vi "Updater Convert TDMS SP Graphics Channel Groups 4.3 to 5.0.vi"(6 "New TDMS File In":refnum<k34>, 8 "error in (no error)":errorcluster, 10 "Group Name In":string, 11 "Source TDMS File In":refnum<k34>) -> (0 "error out":errorcluster, 2 "Group Name Out":string, 3 "Source TDMS File Out":refnum<k34>, 4 "New TDMS File Out":refnum<k34>)   [LabVIEW 2011]
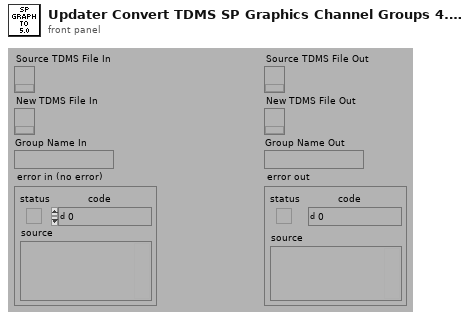
[diagram p1: front panel]
types:
  T1 = typedef "SP Formatting.ctl" = cluster{"Set Format":bool, "Layout":T2, "ActivePlot":i32, "Plots":T3[]}
  T2 = typedef "SP Plot Orientation.ctl" = enum32{"single", "dual", "quad"}
  T3 = typedef "SP Plot.ctl" = cluster{"Orientation":T4, "Ch 1":T5, "Ch 2":T5, "Frequency":cluster{"Start":dbl, "Stop":dbl, "Units":T8, "Override":bool}, "Marker Values":dbl[]}
  T4 = typedef "SP Trace Orientation.ctl" = enum32{"Overlay", "Split"}
  T5 = typedef "SP Display Trace Controls.ctl" = cluster{"Trace On":bool, "Measure":i32, "Format":T6, "Autoscale":bool, "Reference":dbl, "\nRefUnit":string, "Position":dbl, "Scale":dbl, "ScaleUnit":string, "LimitOn":bool, "LimitFill":bool, "Display Data":T7, "Show Markers":bool, "SXX":string}
  T6 = typedef "SP Display Format.ctl" = i32
  T7 = typedef "SP Display Data.ctl" = u16
  T8 = typedef "SP Frequency Units.ctl" = enum16{"Hz", "kHz", "MHz", "GHz", "Points"}
  T9 = typedef "SP Display Parameters.ctl" = cluster{"Lock Control":bool, "Retain Settings":bool, "Formatted Data":bool, "Plot Orientation":enum32{"Single", "Dual", "Quad"}, "Plot Controls":T10[]}
  T10 = typedef "SP Display Plot Controls Cluster.ctl" = cluster{"Trace Orientation":enum32{"Overlay", "Split"}, "Frequency":cluster{"Change Frequency":bool, "Start":dbl, "Stop":dbl, "Units":T8}, "Markers":T11[], "Traces":T5[]}
  T11 = typedef "SP Marker Cluster.ctl" = cluster{"Type":T12, "Frequency (MHz)":dbl}
  T12 = typedef "SP Marker Type.ctl" = enum16{"Frequency", "Trace Maximum", "Trace Minimum", "Limit Maximum", "Limit Minimum"}
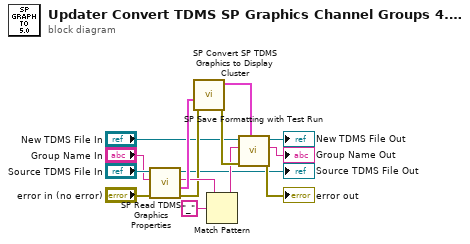
[diagram p0: block diagram]
diagram:
  n1 = call "SP Read TDMS Graphics Properties.vi"("error in (no error)"="error in (no error)", "Group Name In"="Group Name In", "Source TDMS File In"="Source TDMS File In") -> ("error out"=w5:errorcluster, "S Parameter Formatting"=w10:T1, "Group Name Out"=w7:string, "Source TDMS File Out"=→"Source TDMS File Out":refnum<k34>)  [unwired: 5 out]
  n2 = call "SP Convert SP TDMS Graphics to Display Cluster.vi"("error in (no error)"=w5, "S Parameter Formatting"=w10) -> ("error out"=w11:errorcluster, "Display"=w4:T9)  [unwired: 1 in, 7 out]
  n3 = Match Pattern(string=w7, regular expression="_") -> (before substring=w6:string)  [unwired: 4 out]
  n4 = call "SP Save Formatting with Test Run.vi"("Display"=w4, "error in (no error)"=w11, "Group Name In"=w6, "TDMS File Ref In"="New TDMS File In") -> ("error out"=→"error out":errorcluster, "Group Name Out"=→"Group Name Out":string, "TDMS File Ref Out"=→"New TDMS File Out":refnum<k34>)  [unwired: 1 in, 4 out]
